vi "send_data.vi"(8 "error in (no error)":errorcluster, 10 "data":variant, 11 "GenericToplevelComponent in":refnum<class "GenericToplevelComponent.lvclass">) -> (0 "error out":errorcluster, 3 "GenericToplevelComponent out":refnum<class "GenericToplevelComponent.lvclass">, 4 "# elements in queue":i32)   [LabVIEW 2010, in "GenericToplevelComponent.lvclass"]
uses:
  GenericToplevelComponent.lvclass
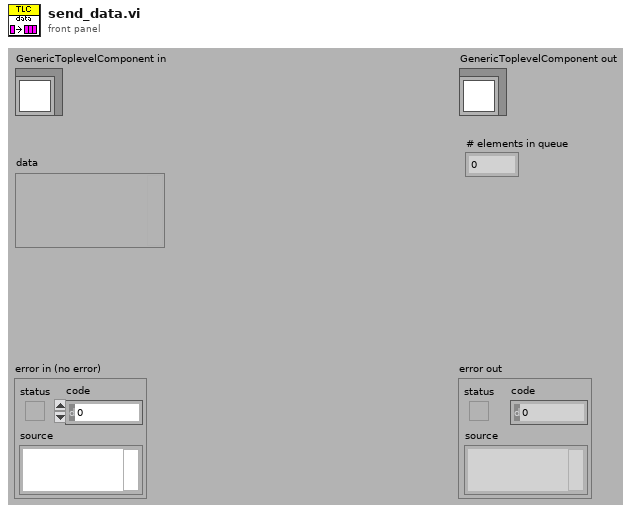
[diagram p1: front panel]
types:
  T1 = typedef "GenericToplevelComponent.lvclass/common_trigger_enum.ctl" = enum16{"NULL", "initialise", "terminate", "fetch command", "fetch data", "attach observer", "register as observer", "detach observer", "acknowledge", "start", "stop", "sweep started", "sweep finished", "experiment started", "experiment stopped"}
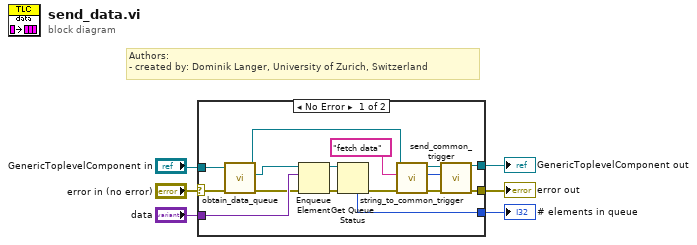
[diagram p0: block diagram]
diagram:
  # "Authors: \n- created by: Dominik Langer, University of Zurich, Switzerland"
  n1 = case shown="No Error" "error in (no error)" {
    selector: "error in (no error)" -> [w18 w24]
    tunnel: [w14 w24] -> w2
    tunnel: [w13 w23] -> w3
    tunnel: "GenericToplevelComponent in" -> [w16 w23]
    tunnel: [w20 _] -> w1
    tunnel: "data" -> [w19 _]
    frame No Error {
      n2 = call-dynamic "obtain_data_queue.vi"("error in (no error)"=w18, "GenericToplevelComponent in"=w16) -> ("error out"=w17:errorcluster, "queue out"=w15:refnum<queue>, "GenericToplevelComponent out"=w10:refnum<class "GenericToplevelComponent.lvclass">)  [unwired: 7 in]
      n3 = Enqueue Element(queue=w15, element=w19, error in (no error)=w17) -> (queue out=w21:refnum<queue>, error out=w22:errorcluster)  [unwired: 2 out]
      n4 = Get Queue Status(queue=w21, error in (no error)=w22) -> (error out=w12:errorcluster, # elements in queue=w20:i32)  [unwired: 7 out]
      n5 = call-dynamic "string_to_common_trigger.vi"("error in (no error)"=w12, "trigger string"="fetch data", "GenericToplevelComponent in"=w10) -> ("error out"=w11:errorcluster, "trigger"=w7:T1, "GenericToplevelComponent out"=w9:refnum<class "GenericToplevelComponent.lvclass">)  [unwired: 6 in]
      n6 = call-dynamic "send_common_trigger.vi"("error in (no error)"=w11, "trigger"=w7, "GenericToplevelComponent in"=w9) -> ("error out"=w14:errorcluster, "GenericToplevelComponent out"=w13:refnum<class "GenericToplevelComponent.lvclass">)  [unwired: 6 in, 1 out]
    }
    frame Error {
    }
  }
  "error out" <- w2
  "GenericToplevelComponent out" <- w3
  "# elements in queue" <- w1
